vi "3.0 EMGtoOMG OFFLINE functional clean.vi"() -> ()   [LabVIEW 2018]
panel:
  in  "Sig 2":bool
  in  "Sig 1":bool
  in  "Sig 3":bool
  out "return value":string
  out "Array":string[](array[string])
  out "c":i32[](array[numeric])
  out "state":dbl[](array[numeric])
  out "charSearch":dbl[](array[numeric])
  out "seq70-104":dbl[](array[numeric])
  out "seq00-34":dbl[](array[numeric])
  out "setID":dbl[](array[numeric])
  out "seq35-69":dbl[](array[numeric])
  in  "stop":bool
  in  "module path":path
  # "1-1-1 -> invalid\n\n1-1-2 -> Set 1 ' abcdeABCDE'\n\n1-1-3 -> Set 2 ' fghijkFGHIJK' \n\n1-2-1 -> Set 3 ' lmnopLMNOP' \n\n1-2-2 -> Set 4 ' qrstuQRSTU'\n\n1-2-3 -> Set 5 ' vwxyzVWXYZ' \n\n1-3-1 -> Set 6 ' .,!>\\'\\\"@#&_-+=' \n\n1-3-2 -> Set 7 ' ()[]<>/\\|%^*~'\n\n1-3-3 -> Set 8 ' 0123456789'"
  # "To the right of the three signals is a \"state\" indicator. \n\nState 1 - \"Unknown\" \n-Program is  waiting for a 1 to start building setID.\n-While in State 1, 2s and 3s don't do anything. \n- Enter a 1 to change to State 2 and begin recording a setID.\n\nState 2 - \"Find\"\n-Program stores next two inputs into setID.\n-The ID can be seen in the setID indicator. The first the numbers is the ID of the set, the 4th number is the associated number of the set (1-8)\n-An ID of 1-1-1 is invalid, and this will change the state back to state 1. \n-All other sets are valid and change state to State 3\n\nState 3 - \"Nav\"\n-Program cycles through and selects a chosen character in a set\n-Repeating 3s will cycle forward through a set, currently selected character is in {}\n-2 will enter the selected character and stay in the current set, and reset the cycle\n-1 will enter the selected character and acts as the first digit in a new setID, and changes to State 2\n\nUse the following sequence as practice:\n2332-121-3-113-3333-122-33333333333-3333-1\n\n2332 does nothing\n121 chooses Set 3\n3 cycles through Set 3\n113 selects character and chooses Set 2\n3333 cycles through Set 2\n122 selects character and chooses Set 4\n33333333333 (eleven 3s) cycles completely through Set 4\n3333 cycles through set 4\n1 selects character"
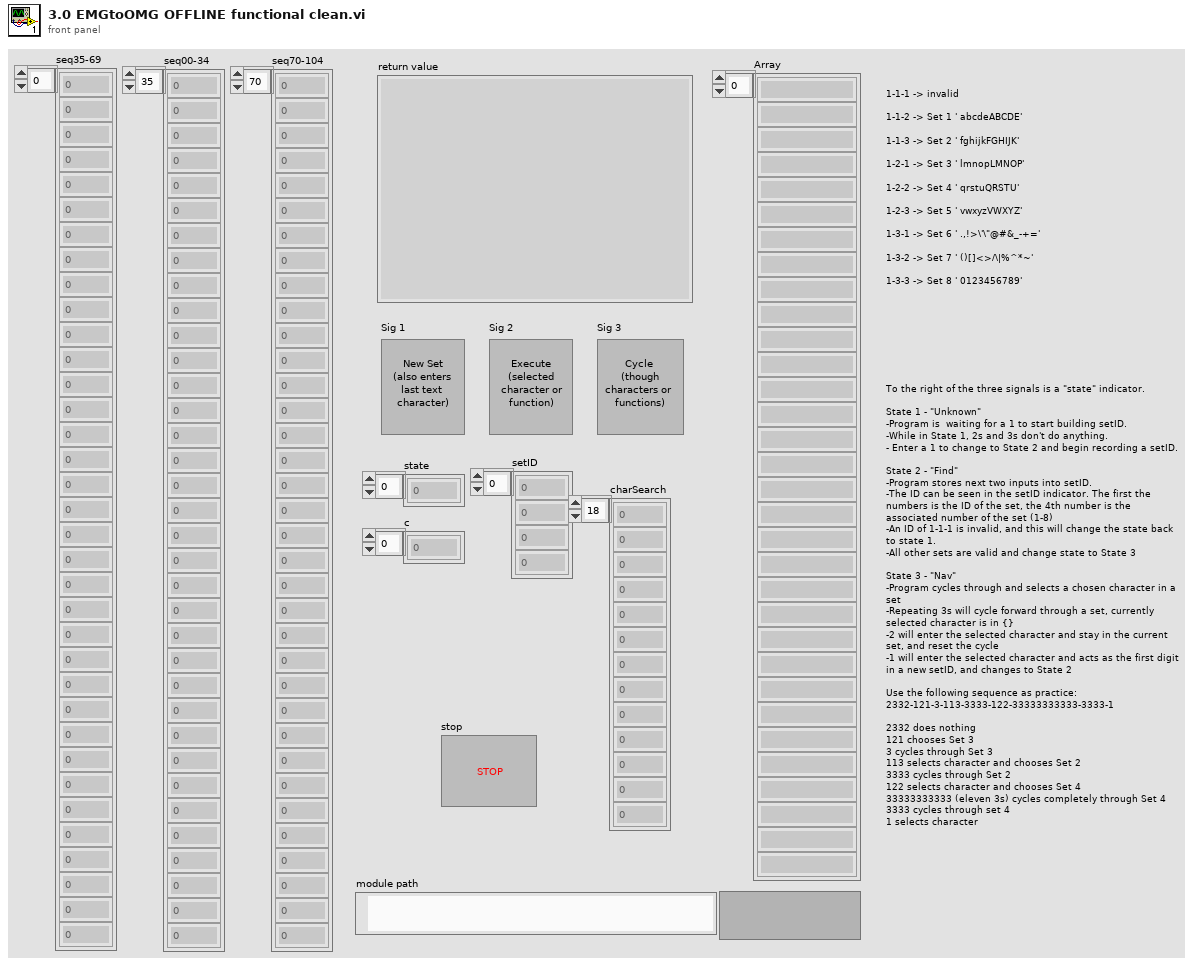
[diagram p1: front panel]
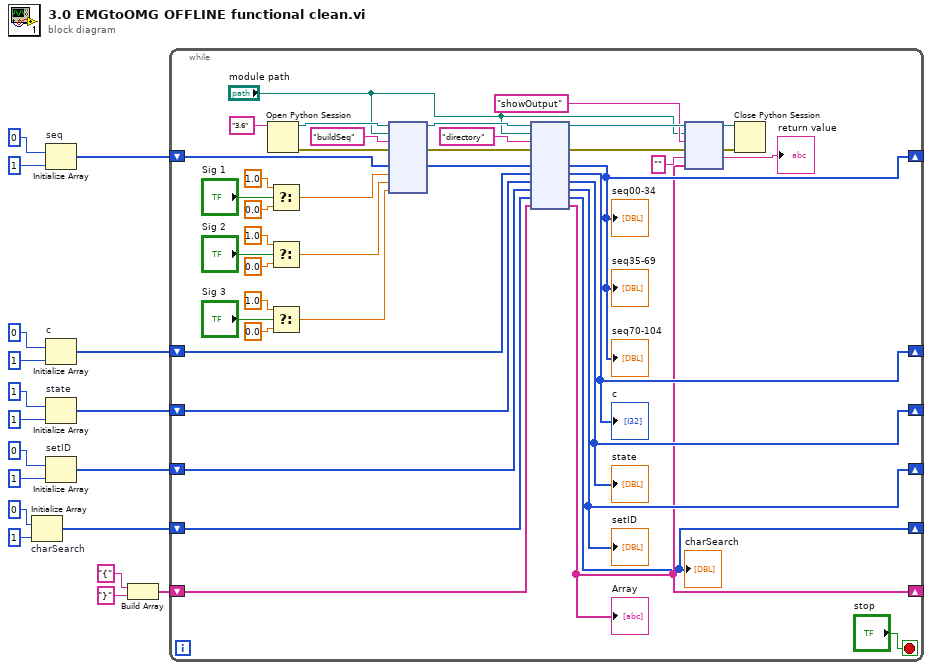
[diagram p0: block diagram]
diagram:
  n1 = Initialize Array "charSearch"(0, 1 ("dimension size")) -> (w13:i32[])
  n2 = Initialize Array "seq"(0, 1 ("dimension size")) -> (w18:i32[])
  n3 = Initialize Array "c"(0, 1 ("dimension size")) -> (w11:i32[])
  n4 = Initialize Array "state"(1, 1 ("dimension size")) -> (w8:i32[])
  n5 = Initialize Array "setID"(0, 1 ("dimension size")) -> (w14:i32[])
  n6 = Build Array("{", "}") -> (w5:string[])
  n7 = while {
    shift-right: [w40] -> _
    shift-left: w18 -> [w51]
    shift-right: [w36] -> _
    shift-left: w14 -> [w39]
    shift-right: [w22] -> _
    shift-left: w13 -> [w38]
    shift-right: [w29] -> _
    shift-left: w5 -> [w37]
    shift-right: [w34] -> _
    shift-left: w8 -> [w35]
    shift-right: [w32] -> _
    shift-left: w11 -> [w33]
    stop <- "stop" stop-if-true
    n8 = Open Python Session(python version="3.6" ("Python version")) -> (session out=w58:refnum<k35>, error out=w57:errorcluster)  [unwired: 2 in]
    n9 = Select(t=1.0, s="Sig 1", f=0.0) -> (s? t:f=w54:dbl)
    n10 = Select(t=1.0, s="Sig 2", f=0.0) -> (s? t:f=w46:dbl)
    n11 = Select(t=1.0, s="Sig 3", f=0.0) -> (s? t:f=w45:dbl)
    n12 = node(w58, "module path", "buildSeq" ("function name"), w57, w51, w54, w46, w45) -> (w44:refnum<k35>, w43:errorcluster, w41:i32[])  [unwired: 5 in, 2 out]
    n13 = node(w44, "module path", "directory" ("function name"), w43, w41, w33, w35, w39, w38, w37) -> (w28:refnum<k35>, w26:errorcluster, w40:i32[], w32:i32[], w34:i32[], w36:i32[], w22:i32[], w29:string[])  [unwired: 2 in, 2 out]
    "seq35-69" <- w40
    "setID" <- w36
    "seq00-34" <- w40
    "seq70-104" <- w40
    "charSearch" <- w22
    "state" <- w34
    "c" <- w32
    "Array" <- w29
    n14 = node(w28, "module path", "showOutput" ("function name"), w26, "", w29) -> (w27:refnum<k35>, w25:errorcluster, →"return value":string)  [unwired: 1 in, 2 out]
    n15 = Close Python Session(session in=w27, error in=w25) -> ()  [unwired: 1 out]
  }
